vi "PCA CreateMaxComponents.vi"(6 "maxComponents":i32, 8 "error in (no error)":errorcluster, 9 "Flags":T1, 10 "Mean":dbl[][](array[numeric]), 11 "Data":dbl[][](array[numeric])) -> (0 "error out":errorcluster, 3 "PCA out":refnum<class "PCA.lvclass">)   [LabVIEW 2020, in "OpenLvVision_OpenCv.lvlib" / "PCA.lvclass"]
doc: "Object by reference!\nThe default constructor initializes an empty PCA structure. The other constructors initialize the structure and call PCA::operator()()"
uses:
  PCA.lvclass
  C:/Users/lukas/Downloads/OpenLvVision_OpenCv/SourceCode/LabView/OpenLvVision_OpenCv/_LvHelpers/EdvrObject/EdvrObject.lvclass
  TypeDef/Flags.ctl
  _LvHelpers/EdvrObject/TypeDef/Edvr.ctl
  _LvHelpers/EdvrObject/EdvrObject.lvclass/EdvrObject.ctl
  _LvHelpers/MatHandling/RegisterMat/RegisterMat_Array2D-DBL.vi
  _LvHelpers/EdvrObject/EdvrObject.lvclass
  OpenLvVision_OpenCv.lvlib
  Dlls/OlvOpenCvWrapper.dll
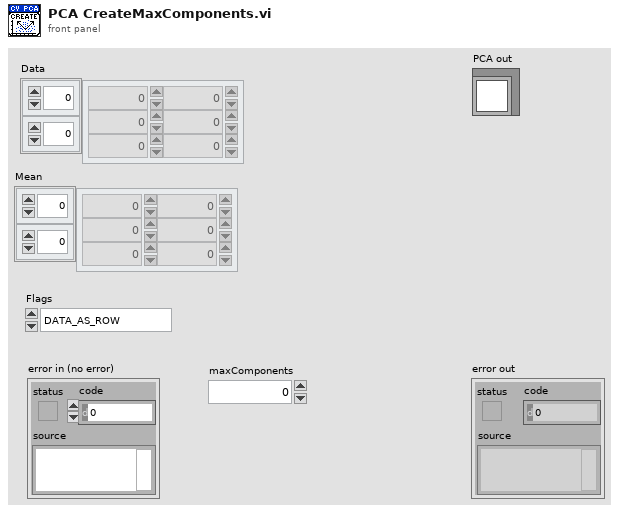
[diagram p1: front panel]
types:
  T1 = typedef "OpenLvVision_OpenCv.lvlib/PCA.lvclass/Flags.ctl" = enum32{"DATA_AS_ROW", "DATA_AS_COL", "USE_AVG"}
  T2 = typedef "OpenLvVision_OpenCv.lvlib/EdvrObject.lvclass/Edvr.ctl" = refnum<data-value>
  T3 = typedef "OpenLvVision_OpenCv.lvlib/MatInfo.ctl" = cluster{"Datatype":T4, "Height":i32, "Width":i32, "Channels":i32, "LineWidth":i32, "Null":u8}
  T4 = typedef "OpenLvVision_OpenCv.lvlib/LvDatatype.ctl" = enum32{"Undefined", "U8", "I8", "U16", "I16", "U32_Color", "I32", "U64_Color", "I64", "SGL", "DBL", "Complex SGL", "Complex DBL", "Array 1D U8", "Array 1D I8", "Array 1D U16", "Array 1D I16", "Array 1D U32_Color", "Array 1D I32", "Array 1D U64_Color", "Array 1D I64", "Array 1D SGL", "Array 1D DBL", "Array 1D Complex SGL", "Array 1D Complex DBL", "Array 2D U8", "Array 2D I8", "Array 2D U16", "Array 2D I16", "Array 2D U32", "Array 2D U32_Color", "Array 2D I32", "Array 2D U64", "Array 2D U64_Color", "Array 2D I64", "Array 2D SGL", "Array 2D DBL", "Array 2D Complex SGL", "Array 2D Complex DBL", "Image Mono U8", "Image Mono U16", "Image Mono I16", "Image Mono SGL", "Image Color U32", "Image Color U64", "ImageComplex Sgl", "Array1d_2dPointI32", "Array1d_2dPointSGL", "Array1d_2dPointDBL", "Array1d_3dPointI32", "Array1d_3dPointSGL", "Array1d_3dPointDBL", "Array1d_4dPointI32", "Array1d_4dPointSGL", "Array1d_4dPointDBL"}
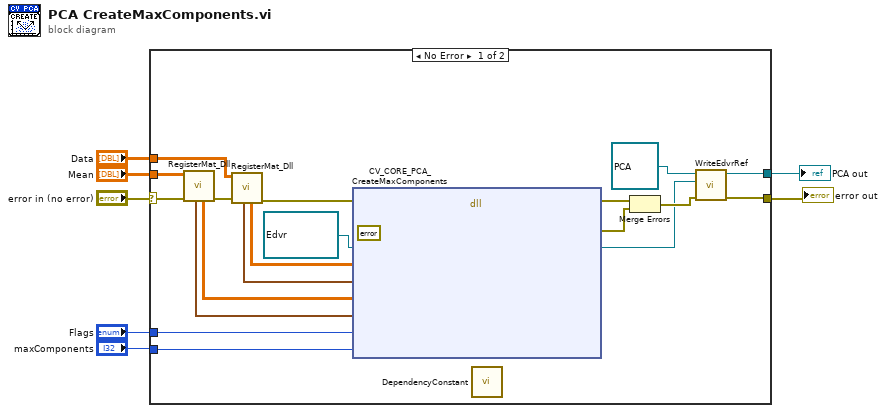
[diagram p0: block diagram]
diagram:
  n1 = case shown="No Error" "error in (no error)" {
    selector: "error in (no error)" -> [w16 w28]
    tunnel: [w26 w28] -> w5
    tunnel: [w27 _] -> w6
    tunnel: "maxComponents" -> [w18 _]
    tunnel: "Flags" -> [w17 _]
    tunnel: "Mean" -> [w15 _]
    tunnel: "Data" -> [w9 _]
    frame No Error {
      n2 = call-poly "RegisterMat_Dll.vi"("error in"=w16, "Array in"=w15) -> ("error out"=w14:errorcluster, "AdressOrData"=w13:dbl[][], "Mat"=w12:T3)  [unwired: 6 in, 1 out]
      n3 = call-poly "RegisterMat_Dll.vi"("error in"=w14, "Array in"=w9) -> ("error out"=w8:errorcluster, "AdressOrData"=w11:dbl[][], "Mat"=w10:T3)  [unwired: 6 in, 1 out]
      n4 = dll-call lib="C:/Users/lukas/Downloads/OpenLvVision_OpenCv/SourceCode/LabView/OpenLvVision_OpenCv/Dlls/OlvOpenCvWrapper.dll" fn="CV_CORE_PCA_CreateMaxComponents"(error in=w8, "Error"=errorcluster {"status"=FALSE, "code"=0, "source"=""} ("error out"), "edvrRef"=T2 refnum ("Edvr"), "addressData"=w11, "matInfoData"=w10, "addressMean"=w13, "matInfoMean"=w12, "flags"=w17, "maxComponents"=w18) -> (error out=w23:errorcluster, "Error"=w20:errorcluster, "edvrRef"=w21:T2)  [unwired: 9 in, 1 out]
      n5 = call "DependencyConstant.vi"() -> ()  [unwired: 12 in]
      n6 = Merge Errors(w23, w20) -> (w22:errorcluster)
      n7 = call "WriteEdvrRef.vi"("error in (no error)"=w22, "Edvr"=w21, "EdvrObject in"=refnum<class "PCA.lvclass"> refnum ("OpenLvVision_OpenCv.lvlib:PCA")) -> ("error out"=w26:errorcluster, "EdvrObject out"=w27:refnum<class "PCA.lvclass">)  [unwired: 7 in]
    }
    frame Error {
    }
  }
  "error out" <- w5
  "PCA out" <- w6
